vi "Initialize command engine state variables.vi"(8 "error in (no error)":errorcluster, 10 "Parameters":T5 {"Compiled"."External Channels"."Channels" format="%.0x"; "Compiled"."External Channels"."Triggers" format="%.0x"}, 11 "Global Variables":T1) -> (0 "error out":errorcluster, 1 "State Variables out":T16, 2 "Parameters out":T5 {"Compiled"."External Channels"."Channels" format="%.0x"; "Compiled"."External Channels"."Triggers" format="%.0x"}, 3 "Global Variables out":T1)   [LabVIEW 2015, in "Instrument Addon Engine.lvlib"]
uses:
  Instrument Addon Engine.lvlib
  Types/command engine global variables.ctl
  <vilib>/NI/AMC/Message Queue.ctl
  <vilib>/NI/AMC/Message.ctl
  <vilib>/NI/Tools/Keyed Array/KeyedArray.ctl
  Types/Commands RT Configuration Cluster.ctl
  Protocols.lvlibp/Protocol Parent/Protocol Parent.lvclass
  Shared/Types/Compiled Settings.ctl
  Shared/Types/Command Parameters.ctl
  Shared/Types/Linked Channel Cluster.ctl
  Shared/Types/Response RT Configuration Cluster.ctl
  Shared/Types/Response Parameters.ctl
  Shared/Types/Response Wait Type.ctl
  Shared/Types/Message Parameters.ctl
  Shared/Types/Message Generation Type.ctl
  Shared/Types/External Trigger Refs.ctl
  <vilib>/NI Veristand/Custom Device API/Data Reference.ctl
  Protections.lvlibp/Parent Protection/Protection.lvclass
  Types/Engine State Variables.ctl
  <vilib>/NI/NIVS Inline Async API/_VS Inline Async API/Process/Process.lvclass
  <vilib>/NI/NIVS Addon Network Comm/Engine/VeriStand Comm.lvclass
  <vilib>/NI/NIVS Inline Async API/_Data Access Engine/Data Access Engine/Types/Write.DVR.ctl
  <vilib>/NI/NIVS Inline Async API/_Data Access Engine/Access Type Classes/Write/Write.lvclass
  <vilib>/NI/NIVS Inline Async API/_Data Access Engine/Data Access Engine/Types/Read.DVR.ctl
  <vilib>/NI/NIVS Inline Async API/_Data Access Engine/Access Type Classes/Read/Read.lvclass
  <vilib>/NI/NIVS Inline Async API/_Data Access Engine/Data Access Engine/Types/ReadWrite.DVR.ctl
  <vilib>/NI/NIVS Inline Async API/_Data Access Engine/Access Type Classes/ReadWrite/ReadWrite.lvclass
  <vilib>/NI/Tools/Keyed Array/Map String.vi
  <vilib>/NI/Tools/String/Get Case Matching.vi
  <vilib>/NI/NIVS Addon Network Comm/Shared/Comm Constants.vi
  <vilib>/NI/Tools/Keyed Array/Tools_KeyedArray.lvlib
  <vilib>/NI/AMC/AMC.lvlib
  <vilib>/NI/NIVS Addon Network Comm/Shared/NI VeriStand Addon Network Comm Shared.lvlib
  Shared/Instrument Addon Shared.lvlib
  <vilib>/NI VeriStand/Custom Device API/Custom Device API.lvlib
  <vilib>/NI/NIVS Inline Async API/_Data Access Engine/Data Access Engine/Data Access Engine.lvclass
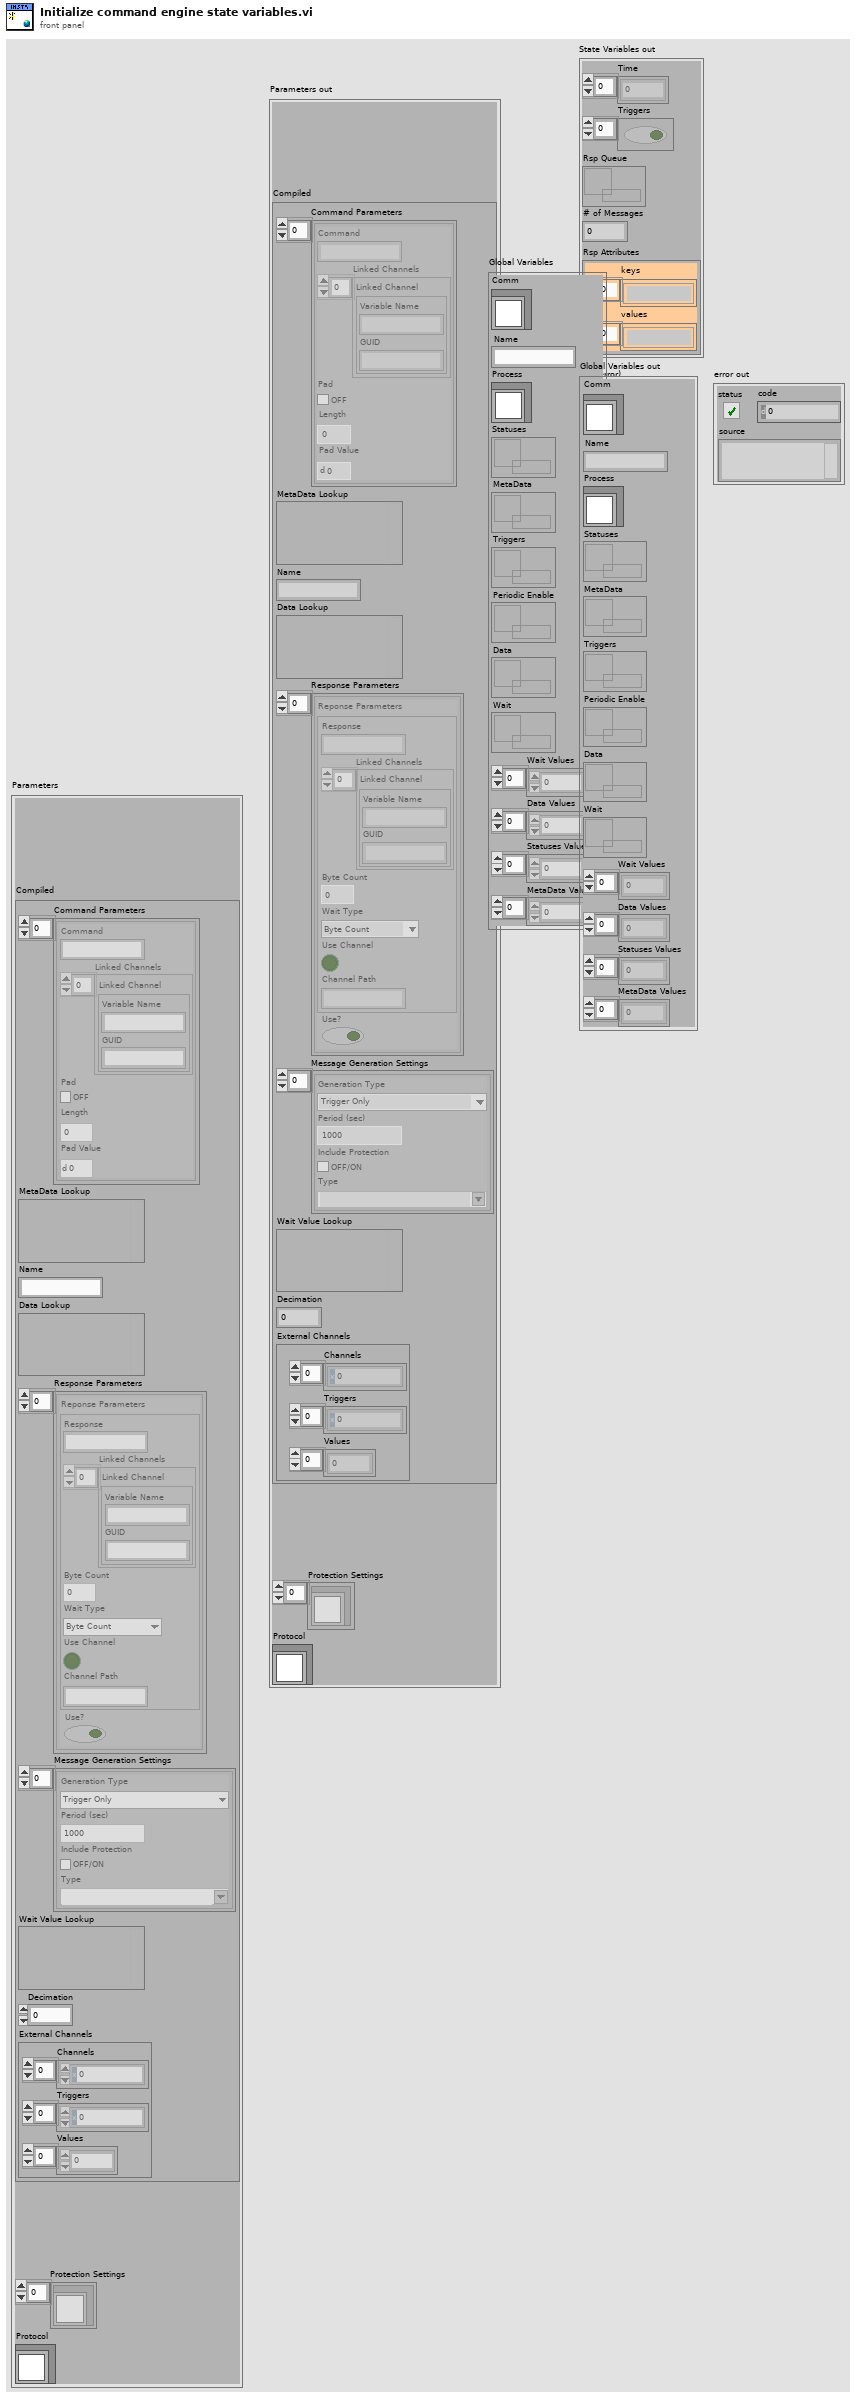
[diagram p1: front panel]
types:
  T1 = typedef "Instrument Addon Engine.lvlib/Engine State Variables.ctl" = cluster{"Comm":refnum<class "VeriStand Comm.lvclass">, "Name":string, "Process":refnum<class "Process.lvclass">, "Statuses":T2, "MetaData":T3, "Triggers":T4, "Periodic Enable":T3, "Data":T2, "Wait":T3, "Wait Values":dbl[], "Data Values":dbl[], "Statuses Values":dbl[], "MetaData Values":dbl[]}
  T2 = typedef "Data Access Engine.lvlib/Data Access Engine.lvclass/Write.DVR.ctl" = refnum<data-value>
  T3 = typedef "Data Access Engine.lvlib/Data Access Engine.lvclass/Read.DVR.ctl" = refnum<data-value>
  T4 = typedef "Data Access Engine.lvlib/Data Access Engine.lvclass/ReadWrite.DVR.ctl" = refnum<data-value>
  T5 = typedef "Instrument Addon Engine.lvlib/Commands RT Configuration Cluster.ctl" = cluster{"Compiled":T6, "Protection Settings":refnum<class "Protection.lvclass">[], "Protocol":refnum<class "Protocol Parent.lvclass">}
  T6 = typedef "Instrument Addon Shared.lvlib/Compiled Settings.ctl" = cluster{"Command Parameters":T7[], "MetaData Lookup":variant, "Name":string, "Data Lookup":variant, "Response Parameters":T9[], "Message Generation Settings":T12[], "Wait Value Lookup":variant, "Decimation":u32, "External Channels":T14}
  T7 = typedef "Instrument Addon Shared.lvlib/Command Parameters.ctl" = cluster{"Command":string, "Linked Channels":T8[], "Pad":bool, "Length":u32, "Pad Value":u8}
  T8 = typedef "Instrument Addon Shared.lvlib/Linked Channel Cluster.ctl" = cluster{"Variable Name":string, "GUID":string}
  T9 = typedef "Instrument Addon Shared.lvlib/Response RT Configuration Cluster.ctl" = cluster{"Reponse Parameters":T10, "Use?":bool}
  T10 = typedef "Instrument Addon Shared.lvlib/Response Parameters.ctl" = cluster{"Response":string, "Linked Channels":T8[], "Type Value":dbl, "Wait Type":T11, "Use Channel":bool, "Channel Path":string}
  T11 = typedef "Instrument Addon Shared.lvlib/Response Wait Type.ctl" = enum16{"Byte Count", "Wait sec"}
  T12 = typedef "Instrument Addon Shared.lvlib/Message Parameters.ctl" = cluster{"Generation Type":T13, "Period":dbl, "Include Protection":bool, "Type":string}
  T13 = typedef "Instrument Addon Shared.lvlib/Message Generation Type.ctl" = enum16{"Trigger Only", "Periodic & Trigger"}
  T14 = typedef "Instrument Addon Shared.lvlib/External Trigger Refs.ctl" = cluster{"Channels":T15[], "Triggers":T15[], "Values":dbl[]}
  T15 = typedef "Custom Device API.lvlib/Data Reference.ctl" = i32
  T16 = typedef "Instrument Addon Engine.lvlib/command engine global variables.ctl" = cluster{"Time":u32[], "Triggers":bool[], "Rsp Queue":T17, "# of Messages":i32, "Rsp Attributes":T18}
  T17 = typedef "AMC.lvlib/Message Queue.ctl" = refnum<queue>
  T18 = typedef "Tools_KeyedArray.lvlib/KeyedArray.ctl" = cluster{"keys":string[], "values":string[]}
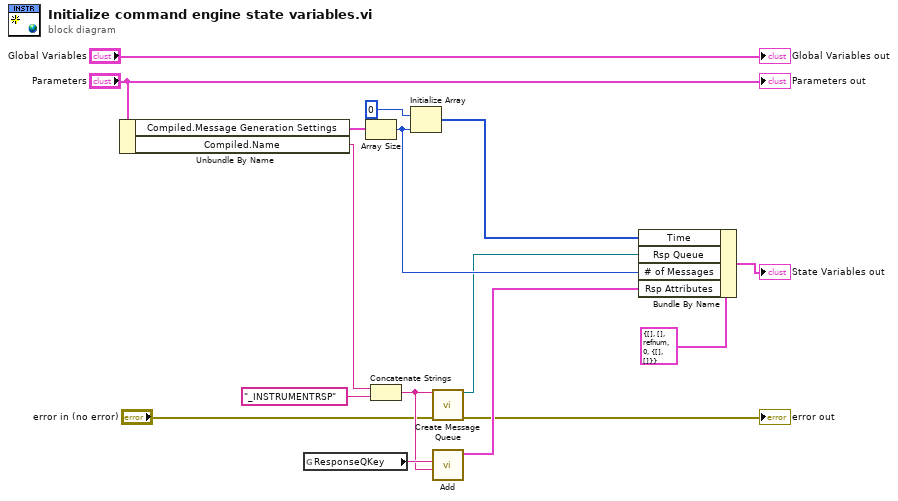
[diagram p0: block diagram]
diagram:
  n1 = Unbundle By Name("Parameters") -> ("Compiled.Message Generation Settings"=w12:T12[], "Compiled.Name"=w8:string)
  n2 = global read "Comm Constants.vi" "ResponseQKey"() -> (w7:string)
  n3 = Array Size(array=w12) -> (size(s)=w15:i32)
  n4 = Concatenate Strings(w8, "_INSTRUMENTRSP" ("message name")) -> (w6:string)
  n5 = Initialize Array(u32 0 ("element"), w15) -> (w14:u32[])
  n6 = call <vilib>:"Create Message Queue.vi"("message queue name"=w6, "error in"="error in (no error)") -> ("message queue out"=w5:T17, "error out"=→"error out":errorcluster)  [unwired: 12 in]
  n7 = call <vilib>:"Add.vi"("value"=w6, "key"=w7) -> ("array out"=w4:T18)  [unwired: 3 in, 2 out]
  n8 = Bundle By Name(cluster=T16 {"Time"=[], "Triggers"=[], "Rsp Queue"=refnum, "# of Messages"=0, "Rsp Attributes"={"keys"=[], "values"=[]}} ("State Variables"), "Time"=w14, "Rsp Queue"=w5, "# of Messages"=w15, "Rsp Attributes"=w4) -> (→"State Variables out":T16)
  "Parameters out" <- "Parameters"
  "Global Variables out" <- "Global Variables"
